vi "Write Associated Cells.vi"(8 "error in (no error)":errorcluster, 10 "Associated Cells":cluster{"PAS":dbl, "CRD":dbl}[](array[cluster]), 11 "Associated Data in":refnum<class "Associated Data.lvclass">) -> (0 "error out":errorcluster, 3 "Associated Data out":refnum<class "Associated Data.lvclass">)   [LabVIEW 2015, in "Associated Data.lvclass"]
uses:
  Associated Data.lvclass
  Associated Data.lvclass/Associated Data.ctl
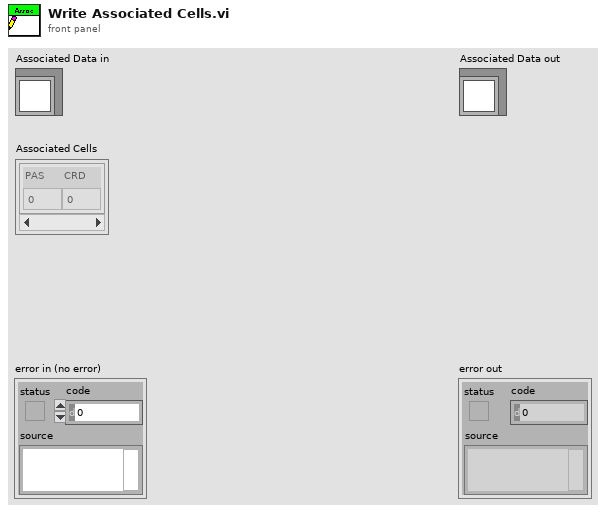
[diagram p1: front panel]
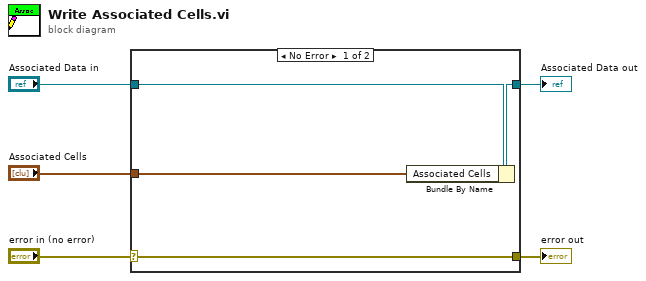
[diagram p0: block diagram]
diagram:
  n1 = case shown="No Error" "error in (no error)" {
    selector: "error in (no error)" -> [w9 w10]
    tunnel: [w9 w10] -> w4
    tunnel: [w7 w11] -> w2
    tunnel: "Associated Data in" -> [w8 w11]
    tunnel: "Associated Cells" -> [w6 _]
    frame No Error {
      n2 = Bundle By Name(cluster=w8, "Associated Cells"=w6) -> (w7:refnum<class "Associated Data.lvclass">)
    }
    frame Error {
    }
  }
  "error out" <- w4
  "Associated Data out" <- w2
